vi "Get SMO PGSQL Log Paths.vi"(5 "getAll Cluster":variant, 7 "Default Paths":string, 8 "error in (no error)":errorcluster, 11 "instrument.PPMS in":refnum<class "instrument.PPMS1.lvclass">) -> (0 "error out":errorcluster, 2 "Paths":string, 3 "instrument.PPMS out":refnum<class "instrument.PPMS1.lvclass">)   [LabVIEW 2019, in "instrument.PPMS1.lvclass"]
uses:
  instrument.PPMS1.lvclass
  instrument.PPMS/instrument.PPMS.lvclass
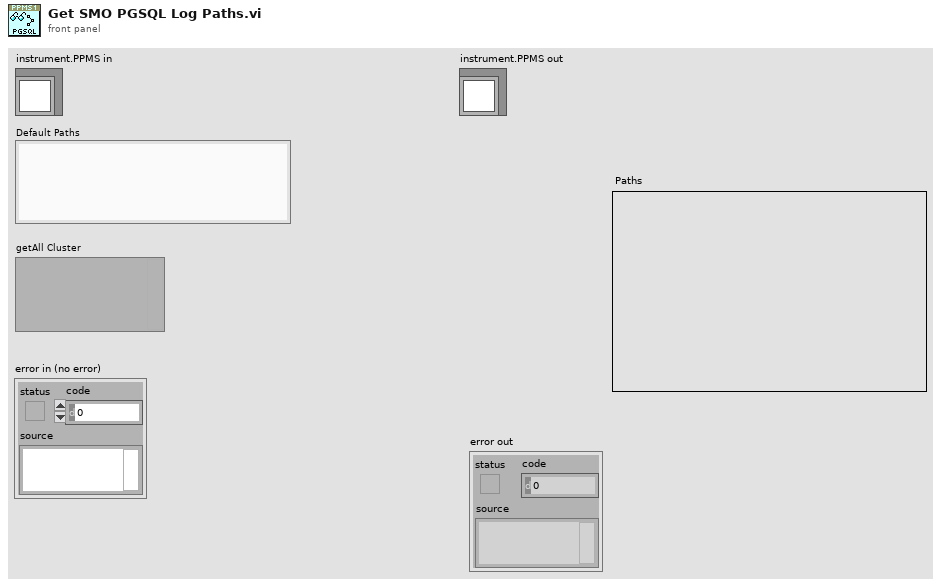
[diagram p1: front panel]
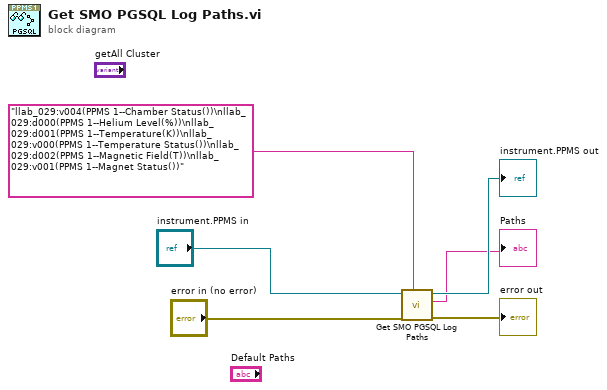
[diagram p0: block diagram]
diagram:
  n1 = call-parent "Get SMO PGSQL Log Paths.vi"("Default Paths"="llab_029:v004(PPMS 1--Chamber Status())\nllab_029:d000(PPMS 1--Helium Level(%))\nllab_029:d001(PPMS 1--Temperature(K))\nllab_029:v000(PPMS 1--Temperature Status())\nllab_029:d002(PPMS 1--Magnetic Field(T))\nllab_029:v001(PPMS 1--Magnet Status())" ("Paths"), "error in (no error)"="error in (no error)", "instrument.PPMS in"="instrument.PPMS in") -> ("error out"=→"error out":errorcluster, "Paths"=→"Paths":string, "instrument.PPMS out"=→"instrument.PPMS out":refnum<class "instrument.PPMS1.lvclass">)  [unwired: 6 in]
